vi "Sub02_BinaryFile.vi"(8 "error in (no error)":errorcluster, 10 "Array":u32[](array[numeric]), 11 "base path":path) -> (0 "error out":errorcluster)   [LabVIEW 2019]
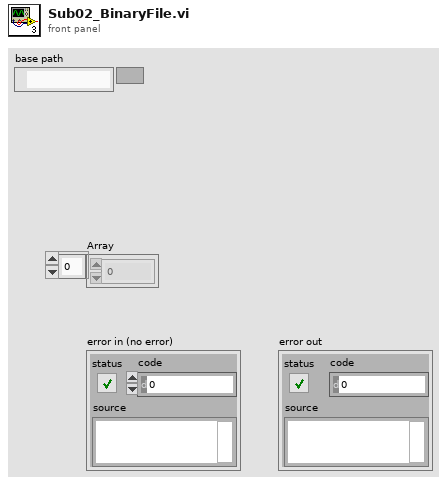
[diagram p1: front panel]
types:
  T1 = enum16{"big-endian, network order", "native, host order", "little-endian"}
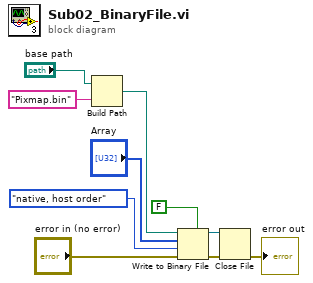
[diagram p0: block diagram]
diagram:
  n1 = Build Path(base path="base path", name or relative path="Pixmap.bin" ("string")) -> (appended path=w3:path)
  n2 = Write to Binary File(file (use dialog)=w3, data="Array", error in="error in (no error)", 5:FALSE ("prepend array or string size? (T)"), 9:T1."native, host order" ("byte order (0:big-endian, network order)")) -> (refnum out=w6:refnum<file>, error out=w7:errorcluster)  [unwired: 1 in, 1 out]
  n3 = Close File(refnum=w6, error in=w7) -> (error out=→"error out":errorcluster)  [unwired: 1 out]
